vi "Global-SystemSettings.vi"() -> ()   [LabVIEW 2013]
panel:
  in  "Database Actor Address":string
  in  "User Name":string
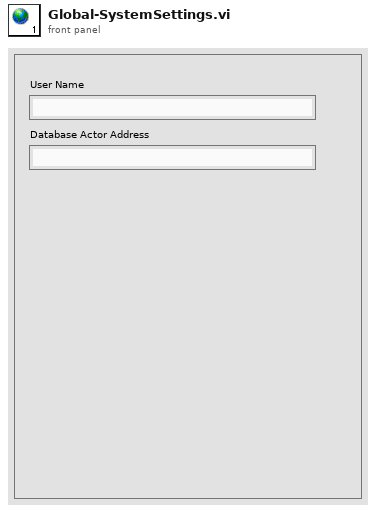
[diagram p1: front panel]
diagram:
